vi "Go To Angle.vi"(8 "error in (no error)":errorcluster, 10 "Angle (°)":dbl, 11 "instrument.PPMS2 in":refnum<class "instrument.PPMS2.lvclass">) -> (0 "error out":errorcluster, 3 "instrument.PPMS2 out":refnum<class "instrument.PPMS2.lvclass">)   [LabVIEW 2016, in "instrument.PPMS2.lvclass"]
uses:
  instrument.PPMS2.lvclass
  PPMS Global.vi
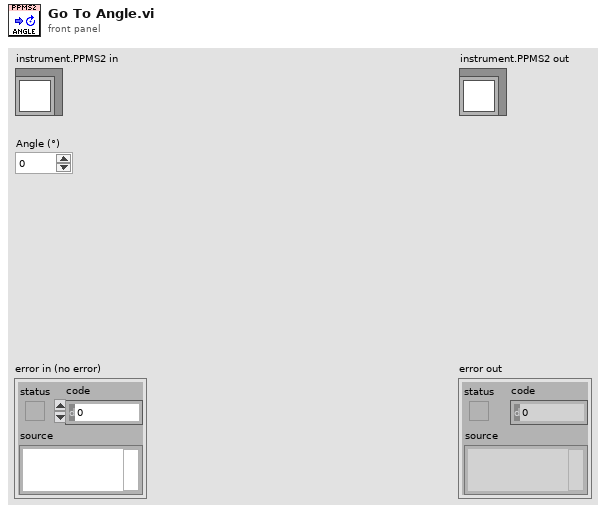
[diagram p1: front panel]
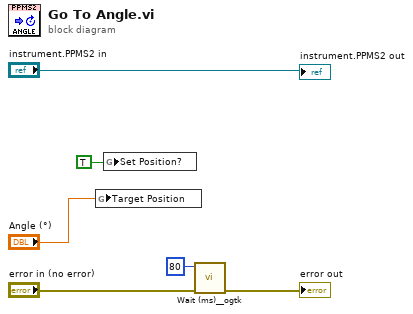
[diagram p0: block diagram]
diagram:
  n1 = global write "PPMS Global.vi" "Target Position"("Angle (°)") -> ()
  n2 = global write "PPMS Global.vi" "Set Position?"(TRUE ("Set Field?")) -> ()
  n3 = call <userlib>:"Wait (ms)__ogtk.vi"("error in (no error)"="error in (no error)", "milliseconds to wait"=u32 80) -> ("error out"=→"error out":errorcluster)  [unwired: 8 in, 1 out]
  "instrument.PPMS2 out" <- "instrument.PPMS2 in"
